vi "Write controlReference.vi"(10 "controlReference":refnum<vi>, 11 "Element in":refnum<class "Element.lvclass">) -> (3 "Element out":refnum<class "Element.lvclass">)   [LabVIEW 2016, in "Element.lvclass"]
uses:
  Element.lvclass
  Element.lvclass/Element.ctl
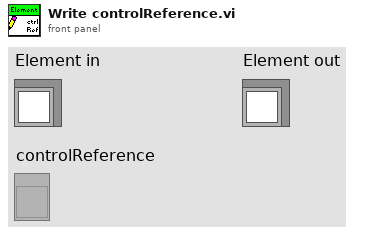
[diagram p1: front panel]
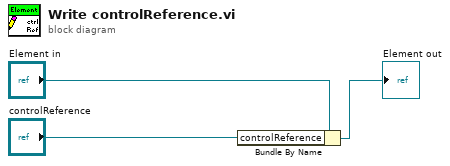
[diagram p0: block diagram]
diagram:
  n1 = Bundle By Name(cluster="Element in", "controlReference"="controlReference") -> (→"Element out":refnum<class "Element.lvclass">)
